vi "deltaMom.vi"(9 "index":i32, 10 "command":T1, 11 "value":dbl) -> (3 "element":dbl)   [LabVIEW 2013]
uses:
  deltaE_FGV_typdef.ctl
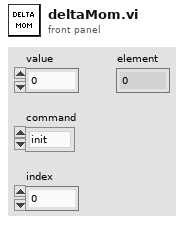
[diagram p1: front panel]
types:
  T1 = typedef "deltaE_FGV_typdef.ctl" = enum16{"init", "set", "read"}
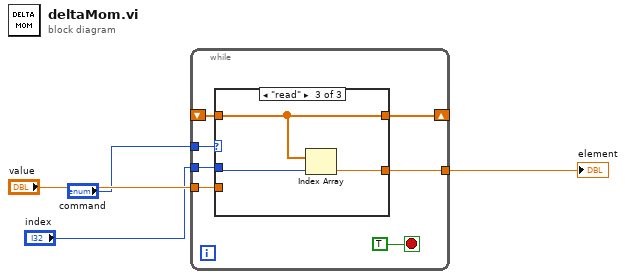
[diagram p0: block diagram]
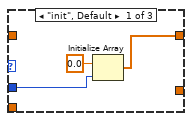
[diagram p2: hidden frame]
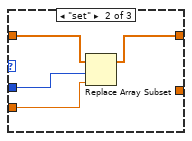
[diagram p3: hidden frame]
diagram:
  n1 = while {
    tunnel: "command" -> [w10]
    shift-right: [w8] -> _
    shift-left: _ -> [w7]
    tunnel: "index" -> [w9]
    tunnel: "value" -> [w6]
    tunnel: [w5] -> w4
    stop <- TRUE stop-if-true
    n2 = case shown="\"read\"" w10 {
      tunnel: w9 -> [w14 w16 w20]
      tunnel: [w12 w15 w21] -> w8
      tunnel: w7 -> [_ w18 w21]
      tunnel: w6 -> [_ w17 _]
      tunnel: [_ _ w19] -> w5
      frame "init", Default {
        n3 = Initialize Array(0.0 ("element"), w14) -> (w12:dbl[])
      }
      frame "set" {
        n4 = Replace Array Subset(array=w18, new element=w17, index=w16) -> (w15:dbl[])
      }
      frame "read" {
        n5 = Index Array(array=w21, index=w20) -> (element=w19:dbl)
      }
    }
  }
  "element" <- w4
